vi "Local Configuration.Transfer Size.Get.vi"(8 "error in (no error)":errorcluster, 11 "GE 5565PIORC":refnum<class "GE 5565PIORC.lvclass">) -> (0 "error out":errorcluster, 2 "Transfer Size":u32, 3 "GE 5565PIORC out":refnum<class "GE 5565PIORC.lvclass">)   [LabVIEW 2016, in "GE 5565PIORC.lvclass"]
uses:
  GE 5565PIORC.lvclass
  GE 5565PIORC.lvclass/GE 5565PIORC.ctl
  <vilib>/Instr/_visa.llb/VISA Register Access Address Space.ctl
  Controls/Registers.Local Configuration.ctl
  Binary Operations/Get Bits U32.vi
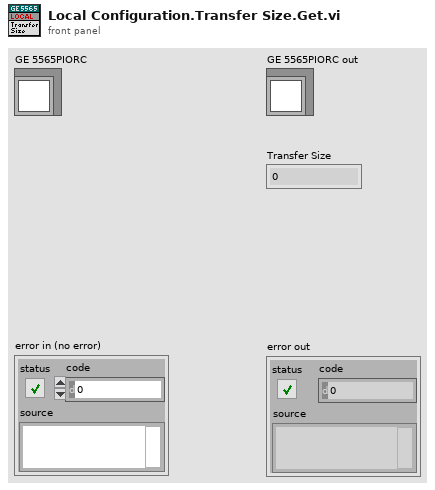
[diagram p1: front panel]
types:
  T1 = typedef "GE 5565PIORC.lvclass/Registers.Local Configuration.ctl" = u32
  T2 = typedef "VISA Register Access Address Space.ctl" = u16
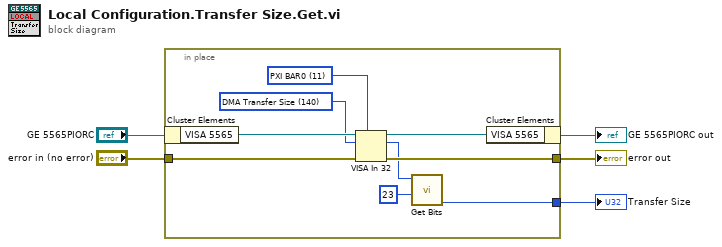
[diagram p0: block diagram]
diagram:
  n1 = in-place {
    in-place-border: "error in (no error)" -> [w12]
    in-place-border: [w11] -> w3
    in-place-border: [w8] -> w1
    w9 = T1 140 items=["INTCSR"=104, "DMA Mode"=128, "DMA PCI Address"=132, "DMA Local Address"=136, "DMA Transfer Size"=140, "DMA Descriptor Pointer"=144, "DMA CSR 0"=168, "DMA PCI DAC Upper Address"=180, "PCI PIO Address Range"=240, "PCI PIO Base Address (Remap)"=244] ("Local Configration Register Offset")
    w10 = T2 11 items=["VXI/VME A16"=1, "VXI/VME A24"=2, "VXI/VME A32"=3, "VXI/VME A64"=4, "PXI Memory Allocations"=9, "PXI Configuration"=10, "PXI BAR0"=11, "PXI BAR1"=12, "PXI BAR2"=13, "PXI BAR3"=14, "PXI BAR4"=15, "PXI BAR5"=16] ("Address Space")
    n2 = in-place-cluster #1("GE 5565PIORC") -> ("VISA 5565"=w14:refnum<visa-resource-name>)
    n3 = VISA In 32(7:w10, 8:w12, 10:w9, 11:w14) -> (0:w11:errorcluster, 2:w7:u32, 3:w13:refnum<visa-resource-name>)
    n4 = call-poly "Get Bits.vi"("Length (1)"=u8 23, "Register in"=w7) -> ("Value"=w8:u32)  [unwired: 6 in, 3 out]
    n5 = in-place-cluster #1("VISA 5565"=w13) -> (→"GE 5565PIORC out":refnum<class "GE 5565PIORC.lvclass">)
  }
  "error out" <- w3
  "Transfer Size" <- w1
